vi "GetBusClass.vi"(8 "ErrorArray In":errorcluster[](array[cluster]), 10 "BusNumber":u8) -> (0 "ErrorArray Out":errorcluster[](array[cluster]), 3 "Framework.lvlib:Bus.lvclass":refnum<class "Bus.lvclass">)   [LabVIEW 2014, in "Bus_class.lvlib" / "Bus.lvclass"]
uses:
  Bus.lvclass
  <vilib>/Utility/error.llb/Error Cluster From Error Code.vi
  <vilib>/ErrorRing/Error Ring.xnode
  <userlib>/NIST/NISTErrorLib/NISTErrorLib.lvlib
  Framework.lvlib
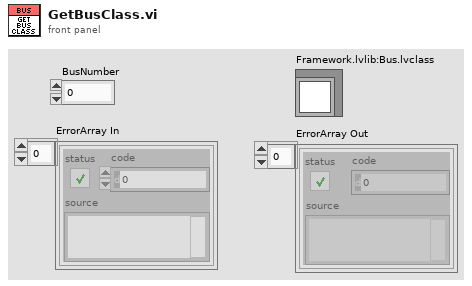
[diagram p1: front panel]
types:
  T1 = typedef "Framework.lvlib/clFrameworkData.ctl" = cluster{"EvtINIFilePaths":path[], "BusClassInstances":refnum<class "Bus.lvclass">[], "PmuImpairINIFilePaths":path[], "FlagImpairINIFilePaths":path[], "NetImpairINIFilePaths":path[], "OutputToFileINIFilePaths":path[], "AppINIFilePaths":path[], "AppModuleID":i32, "OutputToFileID":i32}
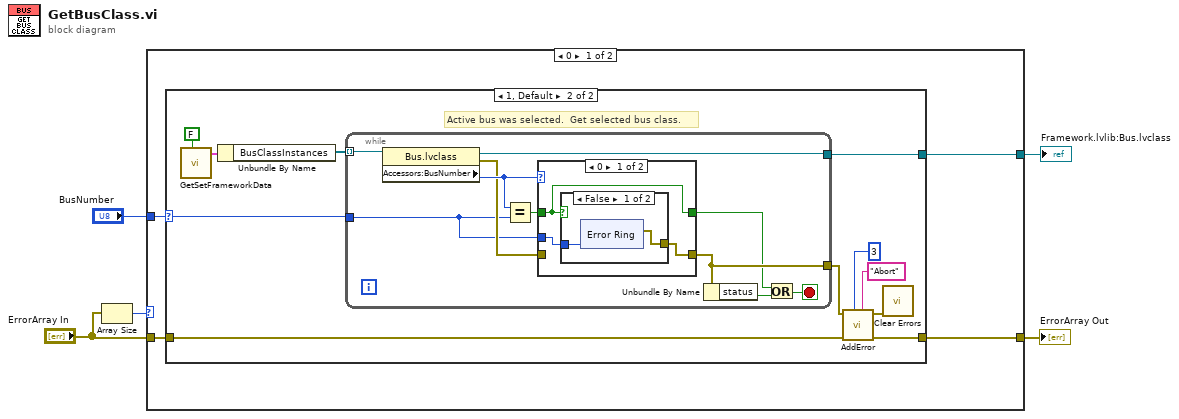
[diagram p0: block diagram]
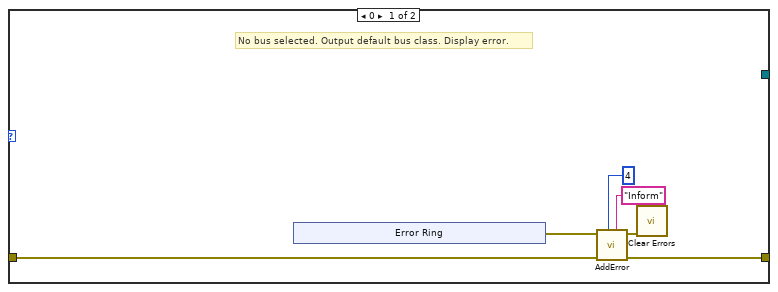
[diagram p2: hidden frame]
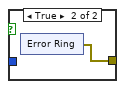
[diagram p3: hidden frame]
diagram:
  n1 = Array Size(array="ErrorArray In") -> (size(s)=w5:i32)
  n2 = case shown="0" w5 {
    tunnel: "ErrorArray In" -> [w8 w62]
    tunnel: [w9 w62] -> w3
    tunnel: [w7 _] -> w2
    tunnel: "BusNumber" -> [w6 _]
    frame 0 {
      n3 = case shown="1, Default" w6 {
        selector: w6 -> [_ w25]
        tunnel: [w11 w31] -> w9
        tunnel: w8 -> [w12 w22]
        tunnel: [_ w24] -> w7
        frame 0 {
          # "No bus selected. Output default bus class. Display error."
          n4 = xnode "Error Ring"() -> ("error out"=w10:errorcluster)
          n5 = call <userlib>:"AddError.vi"("Severity"="Inform" ("String"), "Priority"=u8 4, "ErrorArray"=w12, "error in (no error)"=w10) -> ("ErrorArray"=w11:errorcluster[], "error out"=w15:errorcluster)  [unwired: 6 in]
          n6 = call <vilib>:"Clear Errors.vi"("error in (no error)"=w15) -> ()  [unwired: 5 in, 2 out]
        }
        frame 1, Default {
          # "Active bus was selected.  Get selected bus class."
          n7 = call "GetSetFrameworkData.vi"("Set (F)"=FALSE ("Set/Get")) -> ("clFrameworkData Out"=w26:T1)  [unwired: 10 in]
          n8 = Unbundle By Name(w26) -> ("BusClassInstances"=w23:refnum<class "Bus.lvclass">[])
          n9 = while {
            tunnel: w25 -> [w34]
            tunnel: [w41] -> w24
            tunnel: w23 -> [w40] mode=indexing
            tunnel: [w35] -> w21
            stop <- w38 stop-if-true
            n10 = property class="Bus.lvclass"(reference=w40) -> (reference out=w41:refnum<class "Bus.lvclass">, error out=w36:errorcluster, "Accessors:BusNumber"=w37:u8)  [unwired: 1 in]
            n11 = Equal?(x=w37, y=w34) -> (x = y?=w33:bool)
            n12 = case shown="0" w37 {
              tunnel: [w43 w61] -> w35
              tunnel: w36 -> [_ w61]
              tunnel: w34 -> [w42 _]
              tunnel: w33 -> [w44 w60]
              tunnel: [w44 w60] -> w32
              frame 0 {
                n13 = case shown="False" w44 {
                  tunnel: [w46 w54] -> w43
                  tunnel: w42 -> [w45 _]
                  frame False {
                    n14 = xnode "Error Ring"("parameter 0"=w45) -> ("error out"=w46:errorcluster)
                  }
                  frame True {
                    n15 = xnode "Error Ring"() -> ("error out"=w54:errorcluster)
                  }
                }
              }
              frame 1, Default {
              }
            }
            n16 = Unbundle By Name(w35) -> ("status"=w39:bool)
            n17 = Or(x=w32, y=w39) -> (x .or. y?=w38:bool)
          }
          n18 = call <userlib>:"AddError.vi"("Severity"="Abort" ("String"), "Priority"=u8 3, "ErrorArray"=w22, "error in (no error)"=w21) -> ("ErrorArray"=w31:errorcluster[], "error out"=w30:errorcluster)  [unwired: 6 in]
          n19 = call <vilib>:"Clear Errors.vi"("error in (no error)"=w30) -> ()  [unwired: 5 in, 2 out]
        }
      }
    }
    frame 1, Default {
      # "External error.  Error array holds at least one error."
    }
  }
  "Framework.lvlib:Bus.lvclass" <- w2
  "ErrorArray Out" <- w3
